vi "comm receive bytes.vi"(8 "error in (no error)":errorcluster, 9 "timeout (10000ms)":u32, 10 "no bytes timeout (10ms)":u32, 11 "handle":u64) -> (0 "error out":errorcluster, 1 "received bytes":string, 2 "Byte Count":u32, 3 "dup handle":u64)   [LabVIEW 2009, in "lvserial.lvlib"]
doc: "Reads bytes from serial port until there are no more bytes received during the 'no bytes timeout' or until the timeout value is reached."
uses:
  lvserial.lvlib
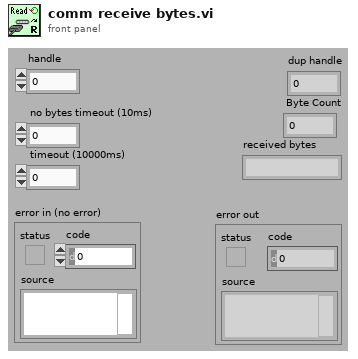
[diagram p1: front panel]
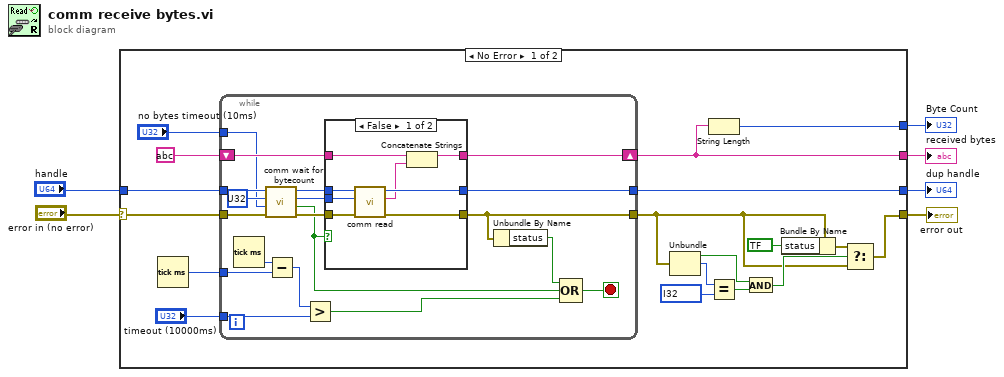
[diagram p0: block diagram]
diagram:
  n1 = case shown="No Error" "error in (no error)" {
    selector: "error in (no error)" -> [w19 w55]
    tunnel: [w23 _] -> w6
    tunnel: "handle" -> [w18 w56]
    tunnel: [w16 w56] -> w5
    tunnel: [w9 w55] -> w1
    tunnel: [w20 _] -> w4
    frame #0 {
      n2 = Tick Count (ms)() -> (millisecond timer value=w22:u32)
      n3 = while {
        tunnel: [w37] -> w16
        tunnel: [w26] -> w8
        tunnel: w19 -> [w36]
        tunnel: "timeout (10000ms)" -> [w39]
        tunnel: w22 -> [w40]
        shift-left: string ? -> [w43]
        shift-right: [w42] -> w20
        tunnel: w18 -> [w35]
        tunnel: "no bytes timeout (10ms)" -> [w30]
        stop <- w28 stop-if-true
        n4 = Tick Count (ms)() -> (millisecond timer value=w41:u32)
        n5 = call "comm wait for bytecount.vi"("error in (no error)"=w36, "timeout (10000)"=w30, "requested byte count"=u32 ?, "Comm Handle"=w35) -> ("error out"=w31:errorcluster, "timed out"=w25:bool, "actual byte count"=w33:u32, "dup Comm Handle"=w32:u64)  [unwired: 1 in, 3 out]
        n6 = Subtract(x=w41, y=w40) -> (x-y=w38:u32)
        n7 = Greater?(x=w38, y=w39) -> (0:w29:bool)
        n8 = case shown="False" w25 {
          tunnel: w43 -> [w51 w53]
          tunnel: [w50 w53] -> w42
          tunnel: [w49 w52] -> w26
          tunnel: [w48 w54] -> w37
          tunnel: w33 -> [w47 _]
          tunnel: w32 -> [w46 w54]
          tunnel: w31 -> [w45 w52]
          frame #0 {
            n9 = call "comm read.vi"("error in (no error)"=w45, "requested byte count"=w47, "Comm Handle"=w46) -> ("error out"=w49:errorcluster, "string read"=w44:string, "dup Comm Handle"=w48:u64)  [unwired: 6 out]
            n10 = Concatenate Strings(w51, w44) -> (w50:string)
          }
          frame #1 {
          }
        }
        n11 = Unbundle By Name(w26) -> ("status"=w27:bool)
        n12 = Compound Arithmetic op=OR(w27, w25, w29) -> (w28:bool)
      }
      n13 = Unbundle(w8) -> ("status"=w12:bool, "code"=w14:i32)  [unwired: 1 out]
      n14 = String Length(string=w20) -> (length=w23:i32)
      n15 = Equal?(x=w14, y=i32 ?) -> (x = y?=w13:bool)
      n16 = And(x=w12, y=w13) -> (x .and. y?=w11:bool)
      n17 = Bundle By Name(cluster=w8, "status"=bool ?) -> (w10:errorcluster)
      n18 = Select(t=w10, s=w11, f=w8) -> (s? t:f=w9:errorcluster)
    }
    frame #1 {
    }
  }
  "dup handle" <- w5
  "Byte Count" <- w6
  "received bytes" <- w4
  "error out" <- w1
